vi "Open Front Panel.vi"(8 "error in (no error)":errorcluster, 9 "state (Standard)":T1(ring)=enum."Standard", 10 "activate? (T)":bool=TRUE, 11 "Protected Actor Handle in":refnum<class "Protected Actor Handle.lvclass">) -> (0 "error out":errorcluster)   [LabVIEW 2020, in "Actor Framework.lvlib" / "Protected Actor Handle.lvclass"]
doc: "Opens the front panel of the running actor's Actor Core clone VI."
uses:
  Protected Actor Handle.lvclass
  Protected Actor Handle.lvclass/Protected Actor Handle.ctl
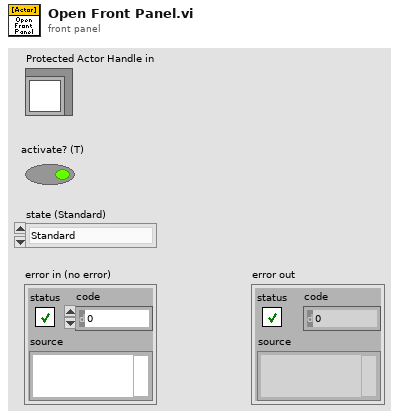
[diagram p1: front panel]
types:
  T1 = enum32{"Invalid", "Standard", "Closed", "Hidden", "Minimized", "Maximized"}
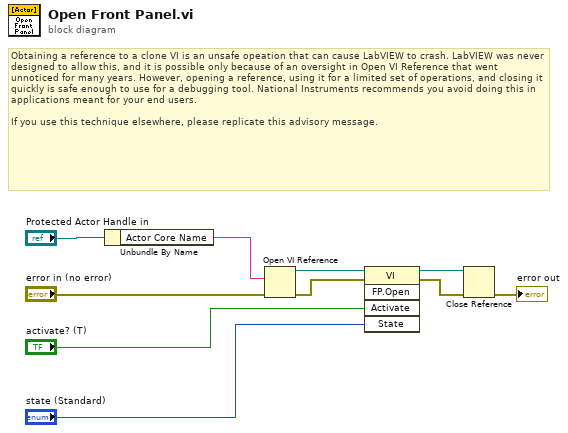
[diagram p0: block diagram]
diagram:
  # "Obtaining a reference to a clone VI is an unsafe opeation that can cause LabVIEW to crash. LabVIEW was never designed to allow this, and it is possible only because of an oversight in Open VI Reference that went unnoticed for many years. However, opening a reference, using it for a limited set of operations, and closing it quickly is safe enough to use for a debugging tool. National Instruments recommends you avoid doing this in applications meant for your end users.\n\nIf you use this technique elsewhere, please replicate this advisory message."
  n1 = Unbundle By Name("Protected Actor Handle in") -> ("Actor Core Name"=w9:string)
  n2 = Open VI Reference(vi path=w9, error in (no error)="error in (no error)") -> (vi reference=w6:refnum<vi>, error out=w5:errorcluster)  [unwired: 4 in]
  n3 = invoke class="VI" method="FP.Open"(reference=w6, error in=w5, "Activate"="activate? (T)", "State"="state (Standard)") -> (reference out=w3:refnum<vi>, error out=w4:errorcluster)  [unwired: 1 in, 3 out]
  n4 = Close Reference(reference=w3, error in (no error)=w4) -> (error out=→"error out":errorcluster)
